vi "AcquireData.vi"(8 "error in (no error)":errorcluster, 11 "923x acquisition config":T4={"NumberOfModules"=0, "Dynamic FPGA VI Ref"=refnum, "KeyphasorX3"=[], "FixedSizeX24"={"EnabledChannels"=[], "Sensitivity"=[], "InputConfig"=[]}, "SamplingInfo"={"Number of Channels"=4, "Sampling Rate"=4.0, "Channels"=[], "Units"=[]}, "BlockSize (sec)"=0.0, "Samples To Read (per chan)"=0, "RunningAcquisitionLength"=0.0, "Settling Time"=0.0, "Waveform Groups"=[], "Acquisition Block Number"=0, "Device Name"="", "ValidConfig"=FALSE} {"FixedSizeX24"."InputConfig" items=["AC Coupled", "DC Coupled", "IEPE AC Coupled"]}) -> (0 "error out":errorcluster, 1 "dataflow messages":T1[](array[typedef]), 3 "923x acquisition config out":T4={"NumberOfModules"=0, "Dynamic FPGA VI Ref"=refnum, "KeyphasorX3"=[], "FixedSizeX24"={"EnabledChannels"=[], "Sensitivity"=[], "InputConfig"=[]}, "SamplingInfo"={"Number of Channels"=4, "Sampling Rate"=4.0, "Channels"=[], "Units"=[]}, "BlockSize (sec)"=0.0, "Samples To Read (per chan)"=0, "RunningAcquisitionLength"=0.0, "Settling Time"=0.0, "Waveform Groups"=[], "Acquisition Block Number"=0, "Device Name"="", "ValidConfig"=FALSE} {"FixedSizeX24"."InputConfig" items=["AC Coupled", "DC Coupled", "IEPE AC Coupled"]}, 5 "settling time requirement met?":bool)   [LabVIEW 2015]
uses:
  <vilib>/addons/InsightCM/Devices/Shared/AcquireBaseLoop/controls/Configuration.ctl
  <vilib>/addons/InsightCM/Devices/Shared/AcquireBaseLoop/controls/TachometerConfig.ctl
  <vilib>/addons/InsightCM/Devices/Shared/AcquireBaseLoop/controls/FixedSizeArrays.ctl
  <vilib>/LabVIEW Targets/FPGA/cRIO/shared/nicrio_ModuleControls/nicrio_cRIO-9232_ConfigModeRing.ctl
  <vilib>/addons/InsightCM/Devices/Shared/cRIOWfmAcq/subVIs/RIO Wfm Cust Ctrls/rwfm_SamplingInfo.ctl
  <vilib>/addons/InsightCM/Devices/Shared/AcquireBaseLoop/controls/Group.ctl
  <vilib>/addons/InsightCM/Devices/Shared/AcquireBaseLoop/controls/Channel.ctl
  <vilib>/addons/InsightCM/Utilities/ChannelStatus/controls/RangeParams.ctl
  <vilib>/addons/InsightCM/Devices/Shared/DataFlow/controls/Data.ctl
  <vilib>/addons/InsightCM/Utilities/DataAccessors/controls/wfmSGL_DVR.ctl
  <vilib>/addons/PointValueMap/controls/PointMap.ctl
  <vilib>/addons/InsightCM/Devices/Shared/AcquireBaseLoop/FpgaAcquisition923x.lvlib
  <vilib>/addons/PointValueMap/PointValueMap.lvlib
  <vilib>/addons/InsightCM/Devices/Shared/DataFlow/DataFlow.lvlib
  <vilib>/addons/InsightCM/Devices/Shared/cRIOWfmAcq/cRIOWfmLib.lvlib
  <vilib>/addons/InsightCM/Utilities/ChannelStatus/ChannelStatus.lvlib
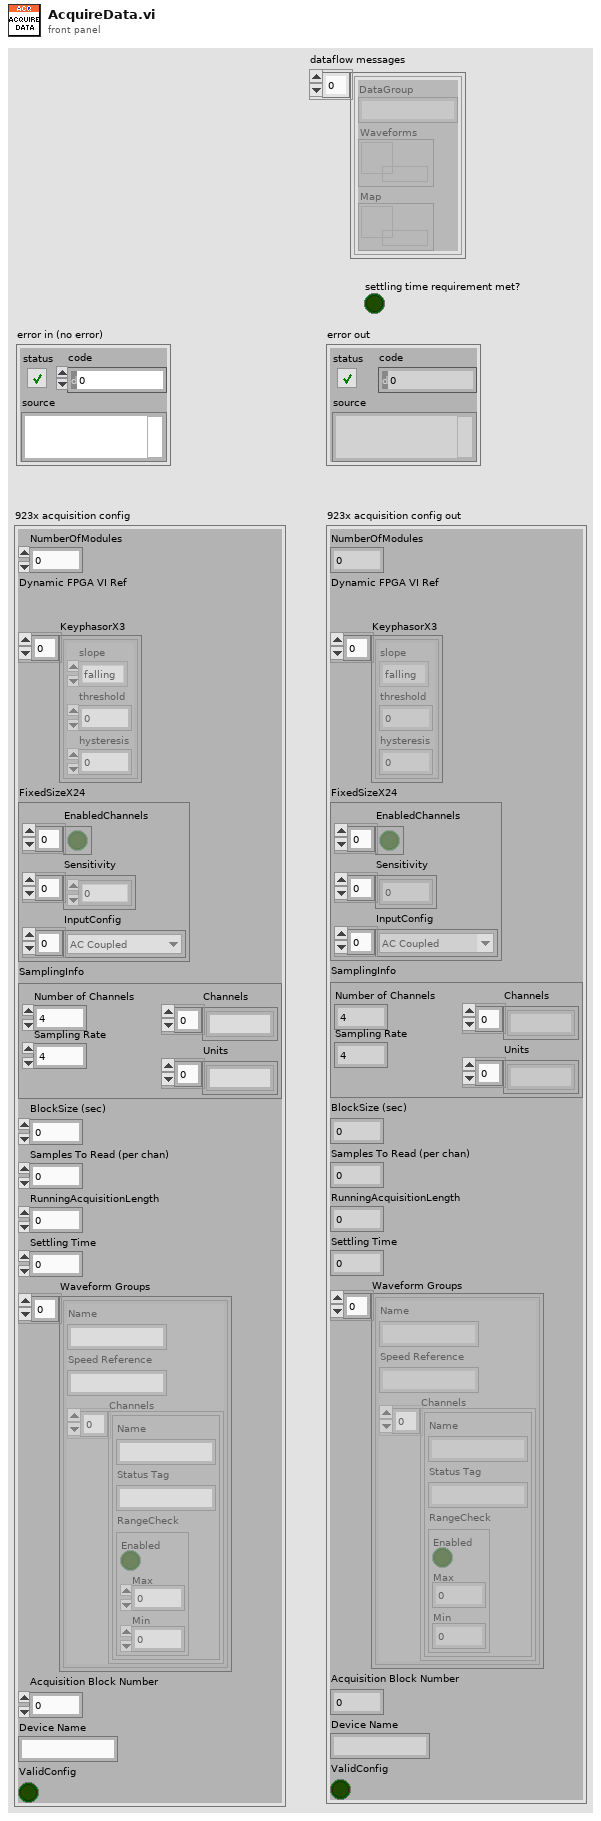
[diagram p1: front panel]
types:
  T1 = typedef "DataFlow.lvlib/Data.ctl" = cluster{"DataGroup":string, "Waveforms":T2, "Map":T3}
  T2 = typedef "wfmSGL_DVR.ctl" = refnum<data-value>
  T3 = typedef "PointValueMap.lvlib/PointMap.ctl" = refnum<data-value>
  T4 = typedef "FpgaAcquisition923x.lvlib/Configuration.ctl" = cluster{"NumberOfModules":i16, "Dynamic FPGA VI Ref":refnum<k20>, "KeyphasorX3":T5[], "FixedSizeX24":T6, "SamplingInfo":T8, "BlockSize (sec)":dbl, "Samples To Read (per chan)":i32, "RunningAcquisitionLength":dbl, "Settling Time":dbl, "Waveform Groups":T9[], "Acquisition Block Number":i32, "Device Name":string, "ValidConfig":bool}
  T5 = typedef "FpgaAcquisition923x.lvlib/TachometerConfig.ctl" = cluster{"slope":enum16{"falling", "rising"}, "threshold":dbl, "hysteresis":dbl}
  T6 = typedef "FpgaAcquisition923x.lvlib/FixedSizeArrays.ctl" = cluster{"EnabledChannels":bool[], "Sensitivity":dbl[], "InputConfig":T7[]}
  T7 = typedef "nicrio_cRIO-9232_ConfigModeRing.ctl" = u8
  T8 = typedef "cRIOWfmLib.lvlib/rwfm_SamplingInfo.ctl" = cluster{"Number of Channels":i32, "Sampling Rate":dbl, "Channels":string[], "Units":string[]}
  T9 = typedef "FpgaAcquisition923x.lvlib/Group.ctl" = cluster{"Name":string, "Speed Reference":string, "Channels":T10[]}
  T10 = typedef "FpgaAcquisition923x.lvlib/Channel.ctl" = cluster{"Name":string, "Status Tag":string, "RangeCheck":T11}
  T11 = typedef "ChannelStatus.lvlib/RangeParams.ctl" = cluster{"Enabled":bool, "Max":dbl, "Min":dbl}
  T12 = typedef "AnalysisHelper.lvlib/PulsePositions.ctl" = cluster{"Name":string, "Pulse Position Data":dbl[], "Pulses Per Rev":i32}
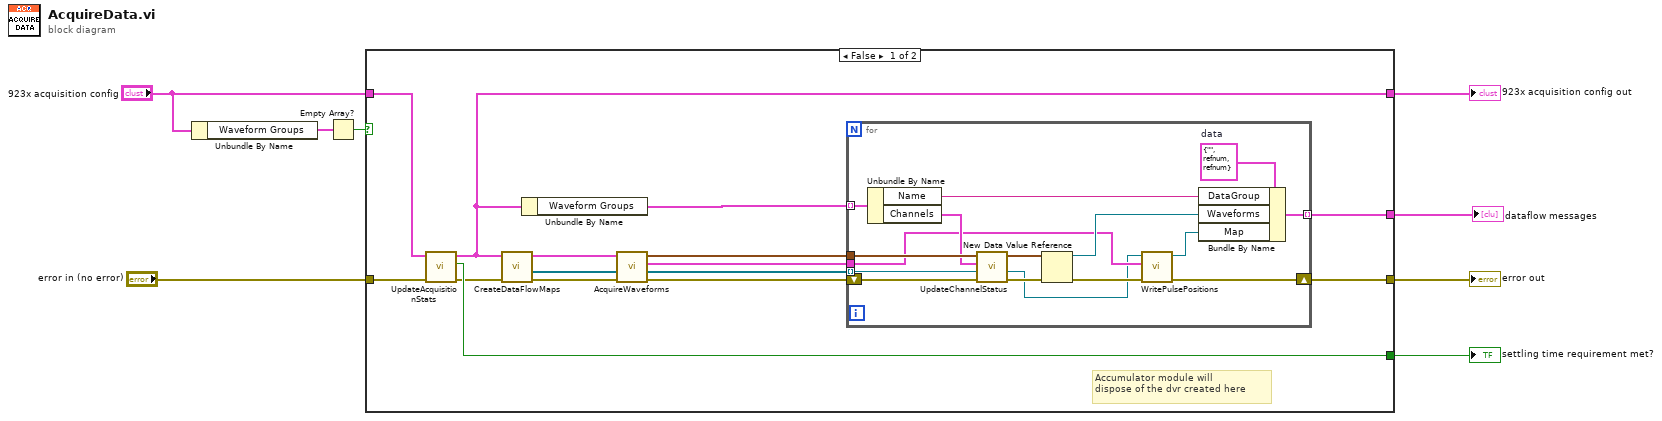
[diagram p0: block diagram]
diagram:
  n1 = Unbundle By Name("923x acquisition config") -> ("Waveform Groups"=w3:T9[])
  n2 = Empty Array?(array=w3) -> (empty?=w1:bool)
  n3 = case shown="False" w1 {
    tunnel: "923x acquisition config" -> [w22 w41]
    tunnel: [w21 _] -> w8
    tunnel: [w19 w41] -> w7
    tunnel: [w14 w40] -> w6
    tunnel: [w13 _] -> w5
    tunnel: "error in (no error)" -> [w12 w40]
    frame False {
      # "Accumulator module will\ndispose of the dvr created here"
      n4 = call <vilib>:"UpdateAcquisitionStats.vi"("error in (no error)"=w12, "configuration"=w22) -> ("error out"=w20:errorcluster, "settling time requirement met?"=w21:bool, "configuration"=w19:T4)  [unwired: 7 in]
      n5 = call <vilib>:"CreateDataFlowMaps.vi"("error in (no error)"=w20, "923x Acquisition Config"=w19) -> ("error out"=w16:errorcluster, "maps"=w18:T3[], "923x Acquisition Config out"=w9:T4)  [unwired: 7 in]
      n6 = Unbundle By Name(w19) -> ("Waveform Groups"=w23:T9[])
      n7 = call "AcquireWaveforms.vi"("error in (no error)"=w16, "Data Flow Maps"=w18, "923x Acquisition Config"=w9) -> ("error out"=w15:errorcluster, "Data Flow Maps out"=w17:T3[], "Pulse Positions Array"=w11:T12[], "Waveforms"=w10:waveform(sgl)[])  [unwired: 2 in, 3 out]
      n8 = for {
        tunnel: w23 -> [w39] mode=indexing
        tunnel: w10 -> [w35]
        tunnel: w11 -> [w27]
        tunnel: w17 -> [w36] mode=indexing
        tunnel: [w38] -> w13 mode=indexing
        shift-right: [w24] -> w14
        shift-left: w15 -> [w37]
        w33 = T1 {"DataGroup"="", "Waveforms"=refnum, "Map"=refnum}  # data
        n9 = Unbundle By Name(w39) -> ("Name"=w32:string, "Channels"=w34:T10[])
        n10 = call <vilib>:"UpdateChannelStatus.vi"("error in (no error)"=w37, "dataflow map in"=w36, "channels"=w34, "acq waveforms"=w35) -> ("error out"=w30:errorcluster, "dataflow map out"=w26:T3, "filtered waveforms"=w31:waveform(sgl)[])  [unwired: 5 in]
        n11 = New Data Value Reference(data value=w31, error in=w30) -> (data value reference=w29:refnum<data-value>, error out=w28:errorcluster)
        n12 = call <vilib>:"WritePulsePositions.vi"("error in (no error)"=w28, "pulse positions array"=w27, "map in"=w26) -> ("error out"=w24:errorcluster, "map out"=w25:T3)  [unwired: 7 in]
        n13 = Bundle By Name(cluster=w33, "DataGroup"=w32, "Waveforms"=w29, "Map"=w25) -> (w38:T1)
      }
    }
    frame True {
    }
  }
  "error out" <- w6
  "settling time requirement met?" <- w8
  "923x acquisition config out" <- w7
  "dataflow messages" <- w5
